vi "WriteToQueue2.vi"(4 "Receiving Data":bool, 6 "Connected":bool, 7 "RxData":string, 8 "error in (no error)":errorcluster, 9 "Consumer State":string, 10 "Producer State":string, 11 "queue":refnum<queue>) -> (0 "error out":errorcluster, 3 "queue out":refnum<queue>)   [LabVIEW 2019]
uses:
  MessageFormat1.ctl
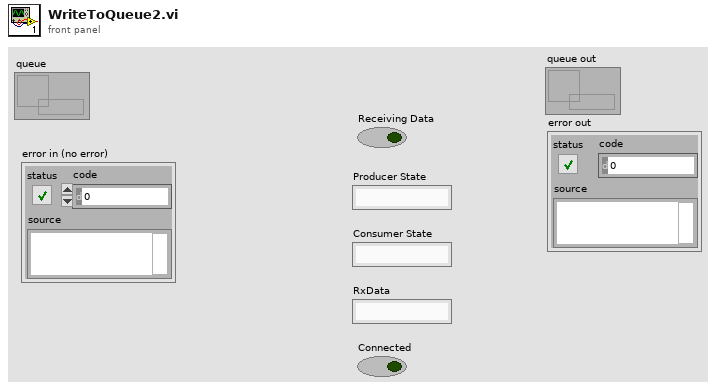
[diagram p1: front panel]
types:
  T1 = typedef "MessageFormat1.ctl" = cluster{"Consumer State":string, "RxData":string, "error constant":errorcluster, "Connected":bool, "Receiving Data":bool, "Producer State ":string}
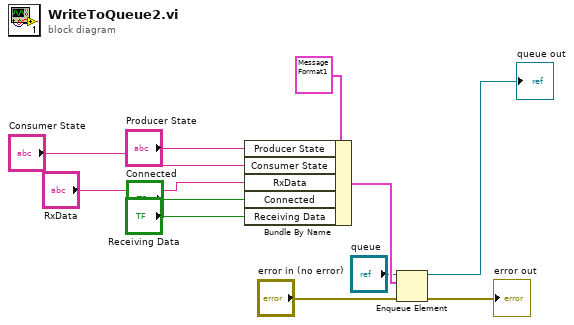
[diagram p0: block diagram]
diagram:
  n1 = Bundle By Name(cluster=T1 {"Consumer State"="Consumer State", "RxData"="Received Data", "error constant"={"status"=FALSE, "code"=0, "source"=""}, "Connected"=FALSE, "Receiving Data"=FALSE, "Producer State "="Producer State"} ("Queue Definition"), "Producer State"="Producer State", "Consumer State"="Consumer State", "RxData"="RxData", "Connected"="Connected", "Receiving Data"="Receiving Data") -> (w6:T1)
  n2 = Enqueue Element(queue="queue", element=w6, error in (no error)="error in (no error)") -> (queue out=→"queue out":refnum<queue>, error out=→"error out":errorcluster)  [unwired: 1 in, 1 out]
